vi "New CycloneDX SBOM.vi"(8 "error in (no error)":errorcluster, 10 "Version (0 = not set)":i32, 11 "Serial number GUID (\"\" = new)":string) -> (0 "error out":errorcluster, 3 "CycloneDX SBOM out":refnum<class "CycloneDX SBOM.lvclass">)   [LabVIEW 2017, in "LabVIEW CycloneDX SBOM.lvlib" / "CycloneDX SBOM.lvclass"]
doc: "Create a new SBOM, setting required/mandatory properties."
uses:
  CycloneDX SBOM.lvclass
  C:/LabVIEW Working Directory/labview-cyclonedx-sbom/Source/CycloneDX/CycloneDX JSON/CycloneDX JSON.lvclass
  CycloneDX JSON/CycloneDX JSON.lvclass
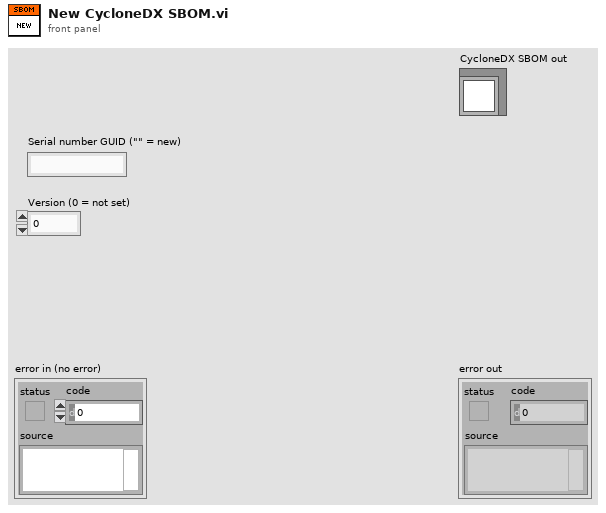
[diagram p1: front panel]
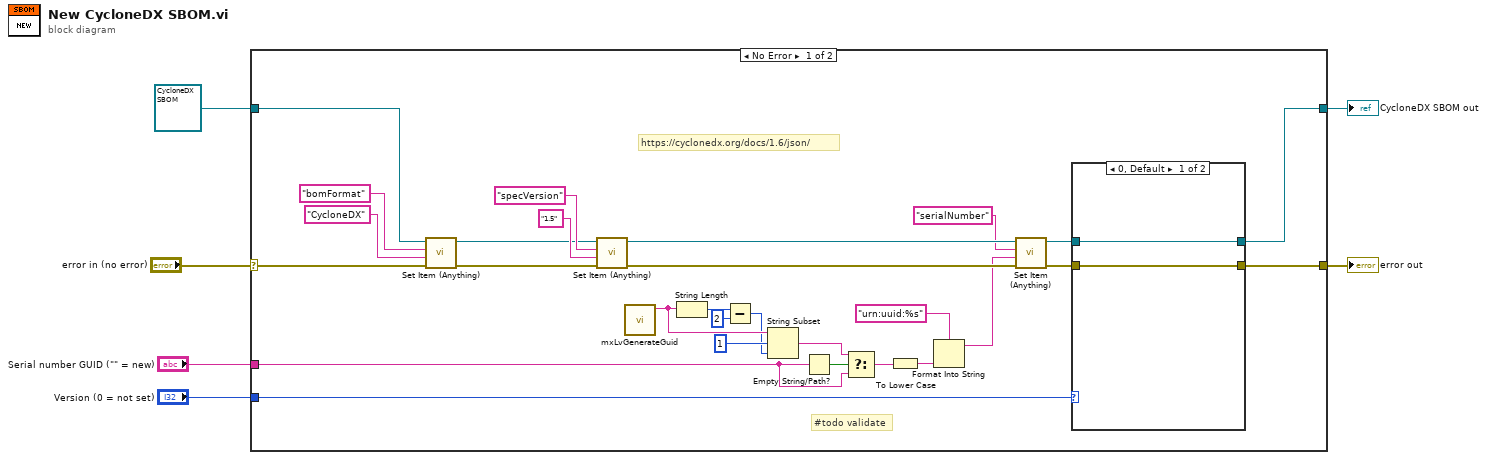
[diagram p0: block diagram]
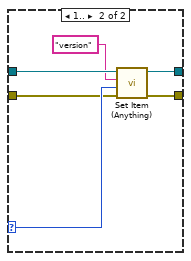
[diagram p2: hidden frame]
diagram:
  n1 = case shown="No Error" "error in (no error)" {
    selector: "error in (no error)" -> [w25 w44]
    tunnel: [w19 w44] -> w5
    tunnel: [w8 w43] -> w3
    tunnel: refnum<class "CycloneDX SBOM.lvclass"> refnum ("CycloneDX SBOM in") -> [w7 w43]
    tunnel: "Version (0 = not set)" -> [w11 _]
    tunnel: "Serial number GUID (\"\" = new)" -> [w24 _]
    frame No Error {
      # "https://cyclonedx.org/docs/1.6/json/"
      # "#todo validate"
      n2 = call "Set Item (Anything).vi"("error in (no error)"=w25, "Value"="CycloneDX" ("Object (or Item) Path"), "Object (or Item) Path"="bomFormat", "CycloneDX SBOM in"=w7) -> ("error out"=w20:errorcluster, "CycloneDX SBOM out"=w16:refnum<class "CycloneDX SBOM.lvclass">)  [unwired: 6 in]
      n3 = call "Set Item (Anything).vi"("error in (no error)"=w20, "Value"="1.5" ("Object (or Item) Path"), "Object (or Item) Path"="specVersion", "CycloneDX SBOM in"=w16) -> ("error out"=w15:errorcluster, "CycloneDX SBOM out"=w13:refnum<class "CycloneDX SBOM.lvclass">)  [unwired: 6 in]
      n4 = call <resource>:"mxLvGenerateGuid.vi"() -> ("Value"=w34:string)  [unwired: 10 in, 1 out]
      n5 = String Length(string=w34) -> (length=w32:i32)
      n6 = Subtract(x=w32, y=2) -> (x-y=w30:i32)
      n7 = String Subset(string=w34, offset (0)=1, length (rest)=w30) -> (substring=w22:string)
      n8 = Empty String/Path?(string/path=w24) -> (empty?=w23:bool)
      n9 = Select(t=w22, s=w23, f=w24) -> (s? t:f=w21:string)
      n10 = To Lower Case(string=w21) -> (all lower case string=w28:string)
      n11 = Format Into String(format string="urn:uuid:%s", w28) -> (resulting string=w14:string)  [unwired: 2 in, 1 out]
      n12 = call "Set Item (Anything).vi"("error in (no error)"=w15, "Value"=w14, "Object (or Item) Path"="serialNumber", "CycloneDX SBOM in"=w13) -> ("error out"=w10:errorcluster, "CycloneDX SBOM out"=w9:refnum<class "CycloneDX SBOM.lvclass">)  [unwired: 6 in]
      n13 = case shown="0, Default" w11 {
        selector: w11 -> [_ w41]
        tunnel: [w36 w42] -> w19
        tunnel: w10 -> [w36 w40]
        tunnel: w9 -> [w35 w39]
        tunnel: [w35 w37] -> w8
        frame 0, Default {
        }
        frame 1.. {
          n14 = call "Set Item (Anything).vi"("error in (no error)"=w40, "Value"=w41, "Object (or Item) Path"="version", "CycloneDX SBOM in"=w39) -> ("error out"=w42:errorcluster, "CycloneDX SBOM out"=w37:refnum<class "CycloneDX SBOM.lvclass">)  [unwired: 6 in]
        }
      }
    }
    frame Error {
    }
  }
  "error out" <- w5
  "CycloneDX SBOM out" <- w3
